vi "SetMatrixSwitch.vi"() -> ()   [LabVIEW 2014]
panel:
  out "String":string
  in  "Array 3":bool[][](array[boolean])
  in  "error in (no error)":errorcluster
  out "error out":errorcluster
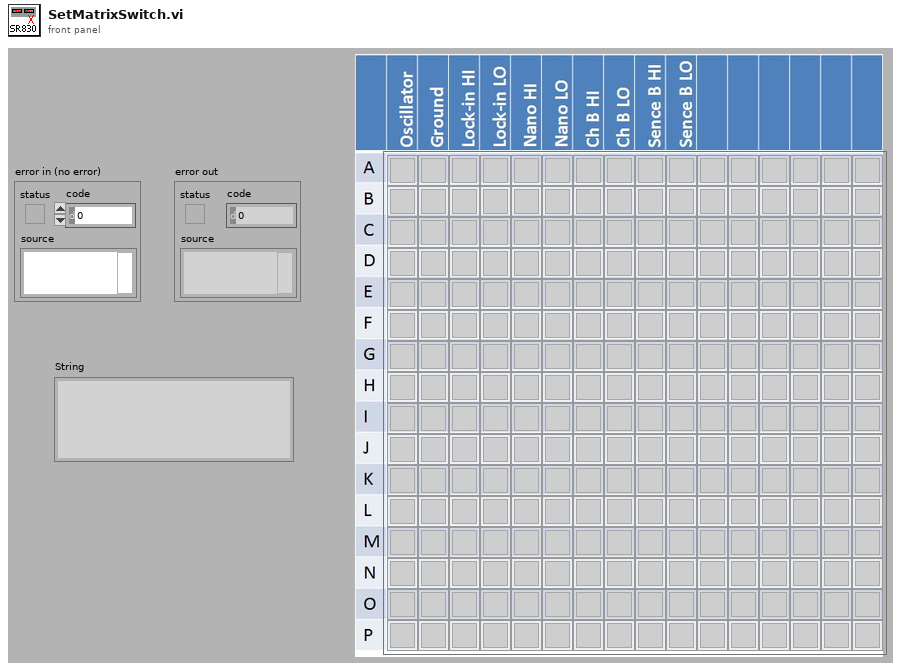
[diagram p1: front panel]
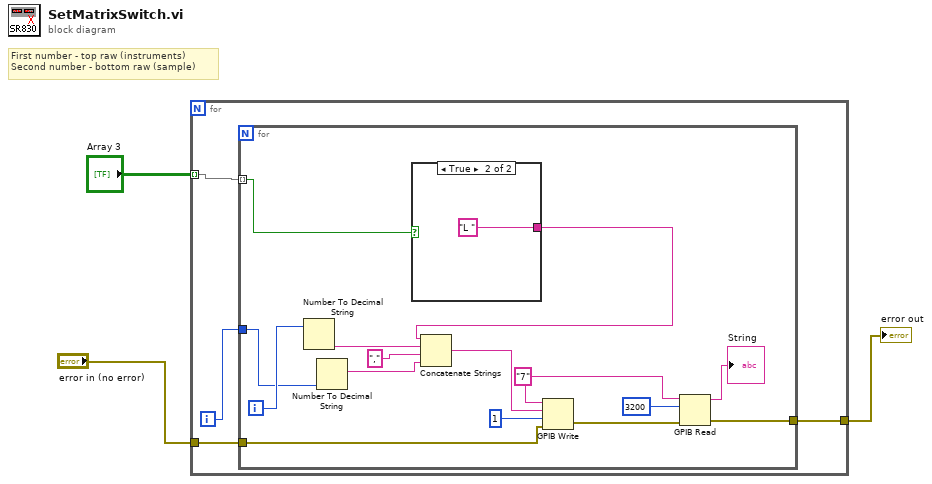
[diagram p0: block diagram]
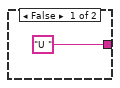
[diagram p2: hidden frame]
diagram:
  # "First number - top raw (instruments)\nSecond number - bottom raw (sample)"
  n1 = for {
    tunnel: [w6] -> w3
    tunnel: "error in (no error)" -> [w5]
    tunnel: "Array 3" -> [w4] mode=indexing
    i -> [w7]
    n2 = for {
      tunnel: w7 -> [w9]
      tunnel: [w13] -> w6
      tunnel: w5 -> [w12]
      tunnel: w4 -> [w8] mode=indexing
      i -> [w10]
      w16 = "7"
      n3 = Number To Decimal String(number=w10) -> (decimal integer string=w21:string)  [unwired: 1 in]
      n4 = Number To Decimal String(number=w9) -> (decimal integer string=w20:string)  [unwired: 1 in]
      n5 = case shown="True" w8 {
        tunnel: ["U " "L "] -> w22
        frame False {
        }
        frame True {
        }
      }
      n6 = Concatenate Strings(w22, w21, ",", w20) -> (w11:string)
      n7 = GPIB Write(0:w16, 1:w11, 2:1, 3:w12) -> (6:w18:errorcluster)  [unwired: 1 in, 1 out]
      n8 = GPIB Read(0:w16, 1:3200, 3:w18) -> (5:→"String":string, 7:w13:errorcluster)  [unwired: 2 in, 1 out]
    }
  }
  "error out" <- w3
